vi "Edit_First_Equal.vi"(1 "String in":string) -> (0 "String out":string)   [LabVIEW 2012]
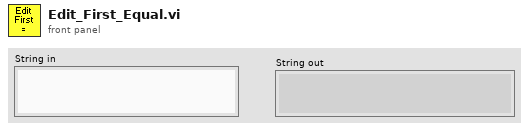
[diagram p1: front panel]
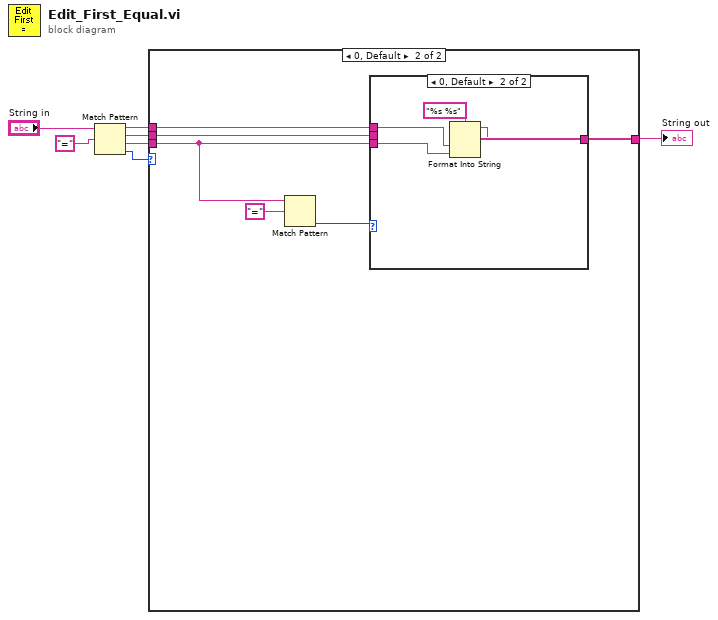
[diagram p0: block diagram]
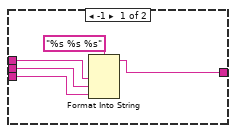
[diagram p3: hidden frame]
diagram:
  n1 = Match Pattern(string="String in", regular expression="=") -> (before substring=w3:string, match substring=w4:string, after substring=w5:string, offset past match=w7:i32)  [unwired: 1 in]
  n2 = case shown="0, Default" w7 {
    tunnel: w3 -> [w8 w14]
    tunnel: w4 -> [_ w13]
    tunnel: w5 -> [_ w11]
    tunnel: [w8 w12] -> w6
    frame -1 {
    }
    frame 0, Default {
      n3 = Match Pattern(string=w11, regular expression="=") -> (offset past match=w9:i32)  [unwired: 1 in, 3 out]
      n4 = case shown="0, Default" w9 {
        tunnel: w14 -> [w19 w23]
        tunnel: w13 -> [w18 _]
        tunnel: [w17 w22] -> w12
        tunnel: w11 -> [w15 w20]
        frame -1 {
          n5 = Format Into String(format string="%s %s %s", w19, w18, w15) -> (resulting string=w17:string)  [unwired: 2 in, 1 out]
        }
        frame 0, Default {
          n6 = Format Into String(format string="%s %s", w23, w20) -> (resulting string=w22:string)  [unwired: 2 in, 1 out]
        }
      }
    }
  }
  "String out" <- w6
